vi "WSVCAP SHL Host TL I2C Write - Multiple Device - Unique Data.vi"(0 "Sub Address [U8]":u8=20 format="%.0x", 11 "error in":errorcluster, 12 "Log (T)":bool=TRUE, 13 "DUT Mask Array (All)":bool[][](array[boolean])=[[TRUE, TRUE, TRUE, TRUE, TRUE, TRUE, TRUE, TRUE, TRUE, TRUE, TRUE, TRUE, TRUE, TRUE, TRUE, TRUE], [TRUE, TRUE, TRUE, TRUE, TRUE, TRUE, TRUE, TRUE, TRUE, TRUE, TRUE, TRUE, TRUE, TRUE, TRUE, TRUE]]) -> (15 "error out":errorcluster)   [LabVIEW 2012]
panel:
  in  "B Data [U8]":u8[](array[numeric]) format="%.0x"
  in  "A Data [U8]":u8[](array[numeric]) format="%.0x"
  out "Socket Mask [U32]":u32=1 format="%08x"
  out "B Data Out":u8[](array[numeric]) format="%.0x"
  out "A Data Out":u8[](array[numeric]) format="%.0x"
  # "DUT 01"
  # "DUT 02"
  # "DUT 03"
  # "DUT 04"
  # "DUT 05"
  # "DUT 06"
  # "DUT 07"
  # "DUT 08"
  # "DUT 09"
  # "DUT 10"
  # "DUT 11"
  # "DUT 12"
  # "DUT 13"
  # "DUT 14"
  # "DUT 15"
  # "DUT 16"
  # "A"
  # "B"
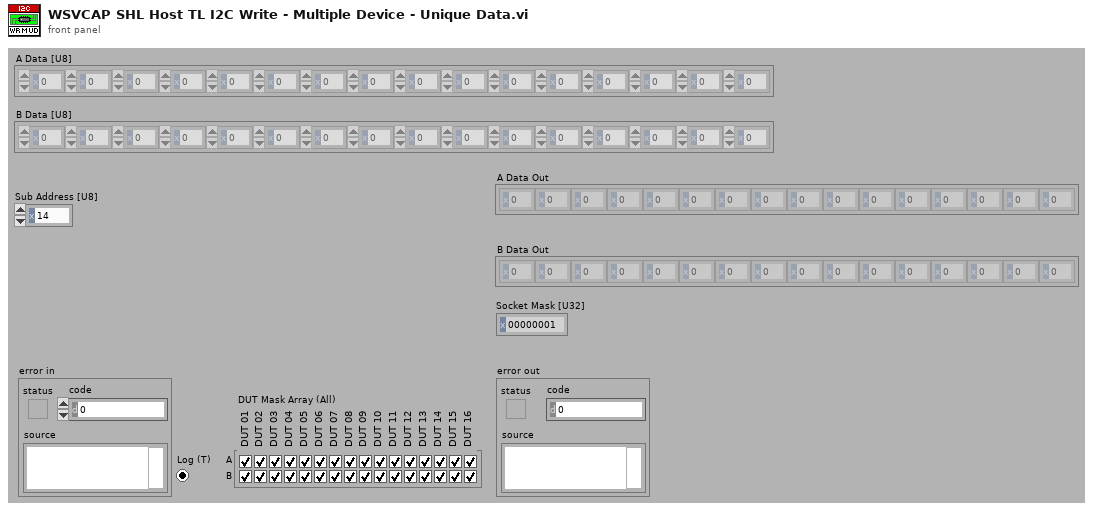
[diagram p1: front panel]
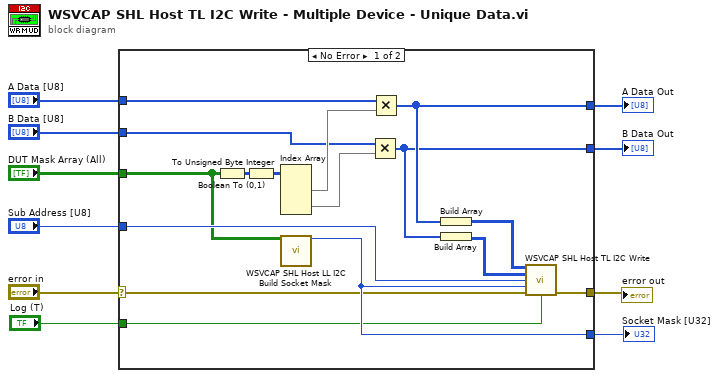
[diagram p0: block diagram]
diagram:
  n1 = case shown="No Error" "error in" {
    selector: "error in" -> [w12 w27]
    tunnel: [w26 w27] -> w10
    tunnel: "Sub Address [U8]" -> [w25 _]
    tunnel: [w15 _] -> w7
    tunnel: [w16 _] -> w6
    tunnel: [w22 _] -> w5
    tunnel: "DUT Mask Array (All)" -> [w21 _]
    tunnel: "A Data [U8]" -> [w14 _]
    tunnel: "B Data [U8]" -> [w13 _]
    tunnel: "Log (T)" -> [w11 _]
    frame No Error {
      n2 = Boolean To (0,1)(Boolean=w21) -> (0, 1=w20:i16[][])
      n3 = To Unsigned Byte Integer(number=w20) -> (unsigned 8bit integer=w17:u8[][])
      n4 = Index Array(array=w17) -> (element #1=w19:u8[], element #2=w18:u8[])  [unwired: 4 in]
      n5 = call "WSVCAP SHL Host LL I2C Build Socket Mask.vi"("DUT Mask Array"=w21) -> ("Socket Mask [U32]"=w22:u32)  [unwired: 13 in, 1 out]
      n6 = Multiply(x=w13, y=w18) -> (x*y=w15:u8[])
      n7 = Multiply(x=w14, y=w19) -> (x*y=w16:u8[])
      n8 = Build Array(w16) -> (w24:u8[][])
      n9 = Build Array(w15) -> (w23:u8[][])
      n10 = call "WSVCAP SHL Host TL I2C Write.vi"("A Data Out"=w24, "B Data Out"=w23, "Sub Address"=w25, "Socket Mask [U32]"=w22, "error in"=w12, "Log (T)"=w11) -> ("error out"=w26:errorcluster)  [unwired: 9 in]
    }
    frame Error {
    }
  }
  "error out" <- w10
  "A Data Out" <- w6
  "B Data Out" <- w7
  "Socket Mask [U32]" <- w5
